vi "Set VISA资源名称.vi"(10 "VISA资源名称":refnum<visa-resource-name>, 11 "DAM0200-Relay in":refnum<class "DAM0200-Relay.lvclass">) -> (3 "DAM0200-Relay out":refnum<class "DAM0200-Relay.lvclass">)   [LabVIEW 2016, in "DAM0200-Relay.lvlib" / "DAM0200-Relay.lvclass"]
uses:
  DAM0200-Relay.lvclass
  DAM0200-Relay.lvclass/DAM0200-Relay.ctl
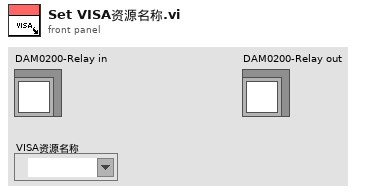
[diagram p1: front panel]
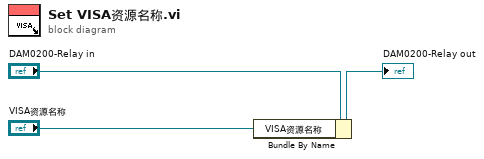
[diagram p0: block diagram]
diagram:
  n1 = Bundle By Name(cluster="DAM0200-Relay in", "VISA资源名称"="VISA资源名称") -> (→"DAM0200-Relay out":refnum<class "DAM0200-Relay.lvclass">)
